vi "Check Stream Status.vi"(0 "niUsrpRio Session":T1={"FPGA Interface"=refnum, "RIO Interface Number"=0, "Data Clock Rate"=0, "FPGA Data Clock Rate"=0, "Global Settings Register Bus"=refnum, "Radio 0 Settings Register Bus"=refnum, "Radio 1 Settings Register Bus"=refnum, "Radio Settings Bus Semaphore"=refnum, "DB Queues"=[], "Characterization Data Valid?"=FALSE, "EEPROM Header"={"Checksum"=0, "Product Code"=0, "Hardware Current Version"=0, "Hardware Oldest Compatible Version"=0, "EEPROM Map Current Version"=0, "EEPROM Map Oldest Compatible Version"=0, "User Password"="", "Pointer to Factory Header"=0, "Pointer to User Header"=0, "Recommended Interval"=0, "Number of Reserved Bytes"=9, "Number of Daughterboards"=0, "Daughterboard IDs"=[], "Daughterboard Serial Numbers"=[]}, "Device Data Header"={"Checksum"=0, "Number of Channels"=0, "Number of Gain Settings"=[], "Pointer to Characterization Data"=[], "Number of Reserved Bytes"=27, "Number of Frequencies"=[]}, "EEPROM Characterization Header"={"Checksum"=0, "Date"=timestamp(0 s since 1904-01-01), "Temperature"=0.0, "Misc. Info"="", "Pointer to Device Data Header"=0, "Number of Reserved Bytes"=28}, "Characterization Data"=[], "FPGA Current Version"=0, "FPGA Oldest Compatible Version"=0, "Fixed Logic Current Version"=0, "Fixed Logic Oldest Compatible Version"=0, "FPGA Radio Settings Bus Current Version"=0, "FPGA Radio Settings Bus Oldest Compatible Version"=0, "FPGA Board Config Current Version"=0, "FPGA Board Config Oldest Compatible Version"=0} {"FPGA Data Clock Rate" format="%#.3pHz"; "Data Clock Rate" format="%#.3pHz"; "Characterization Data"."Frequencies [Hz]" format="%#_6p"; "EEPROM Characterization Header"."Pointer to Device Data Header" format="%x"; "EEPROM Characterization Header"."Checksum" format="%x"; "Device Data Header"."Pointer to Characterization Data" format="%x"; "Device Data Header"."Checksum" format="%x"; "EEPROM Header"."Pointer to User Header" format="%x"; "EEPROM Header"."Pointer to Factory Header" format="%x"; "EEPROM Header"."Product Code" format="%x"; "EEPROM Header"."Checksum" format="%x"}, 1 "scope":string(combo)="rx", 11 "error in":errorcluster, 12 "reference frequency source":string(combo)="Internal" caption="Reference Frequency Source") -> (4 "niUsrpRio Session (out)":T1={"FPGA Interface"=refnum, "RIO Interface Number"=0, "Data Clock Rate"=0, "FPGA Data Clock Rate"=0, "Global Settings Register Bus"=refnum, "Radio 0 Settings Register Bus"=refnum, "Radio 1 Settings Register Bus"=refnum, "Radio Settings Bus Semaphore"=refnum, "DB Queues"=[], "Characterization Data Valid?"=FALSE, "EEPROM Header"={"Checksum"=0, "Product Code"=0, "Hardware Current Version"=0, "Hardware Oldest Compatible Version"=0, "EEPROM Map Current Version"=0, "EEPROM Map Oldest Compatible Version"=0, "User Password"="", "Pointer to Factory Header"=0, "Pointer to User Header"=0, "Recommended Interval"=0, "Number of Reserved Bytes"=9, "Number of Daughterboards"=0, "Daughterboard IDs"=[], "Daughterboard Serial Numbers"=[]}, "Device Data Header"={"Checksum"=0, "Number of Channels"=0, "Number of Gain Settings"=[], "Pointer to Characterization Data"=[], "Number of Reserved Bytes"=27, "Number of Frequencies"=[]}, "EEPROM Characterization Header"={"Checksum"=0, "Date"=timestamp(0 s since 1904-01-01), "Temperature"=0.0, "Misc. Info"="", "Pointer to Device Data Header"=0, "Number of Reserved Bytes"=28}, "Characterization Data"=[], "FPGA Current Version"=0, "FPGA Oldest Compatible Version"=0, "Fixed Logic Current Version"=0, "Fixed Logic Oldest Compatible Version"=0, "FPGA Radio Settings Bus Current Version"=0, "FPGA Radio Settings Bus Oldest Compatible Version"=0, "FPGA Board Config Current Version"=0, "FPGA Board Config Oldest Compatible Version"=0} {"FPGA Data Clock Rate" format="%#.3pHz"; "Data Clock Rate" format="%#.3pHz"; "Characterization Data"."Frequencies [Hz]" format="%#_6p"; "EEPROM Characterization Header"."Pointer to Device Data Header" format="%x"; "EEPROM Characterization Header"."Checksum" format="%x"; "Device Data Header"."Pointer to Characterization Data" format="%x"; "Device Data Header"."Checksum" format="%x"; "EEPROM Header"."Pointer to User Header" format="%x"; "EEPROM Header"."Pointer to Factory Header" format="%x"; "EEPROM Header"."Product Code" format="%x"; "EEPROM Header"."Checksum" format="%x"}, 6 "done":bool caption="Done", 15 "error out":errorcluster)   [LabVIEW 2015]
doc: "Checks the status of the stream for when it is done, for FIFO overflows, for FIFO underflows, for DSP overflows, and if the clocks ever became unlocked. Checks the stream status after each Fetch Rx Data/Write Tx Data.\n\n<B>Input Parameters</B>\n\n<B>niUsrpRio Session</B> is the object created by the Open VI and used as the session handle for the USRP RIO design library.\n\n<B>Reference Frequency Source</B> is used when the source is GPS to determine whether to check whether the GPS became unlocked.\n\n<B>scope</B> is the channel to check the stream status. The options are \"rx/RF 0\", \"rx/RF 1\", \"tx/RF 0\", and \"tx/RF 1\".\n\n<B>error in</B> describes error conditions that occur before this node runs. This input provides standard 'error in' functionality.\n\n<B>Output Parameters</B>\n\n<B>niUsrpRio Session (out)</B> is the niUsrpRio session used in all subsequent USRP RIO design library host VIs.\n\n<B>Done</B> indicates when the acquisition/generation has completed.\n\n<B>error out</B> contains error information. This output provides standard 'error out' functionality."
uses:
  <instrlib>/niUsrpRio/Config/v1/Host/Public/niUsrpRio Session.ctl
  <instrlib>/_niInstr/Register Bus/v0/Host/Public/Register Bus Session.ctl
  <instrlib>/_niInstr/Register Bus/v0/Host/Private/Session Data.ctl
  <instrlib>/niUsrpRio/Config/v1/Host/Private/DB Queue Reference.ctl
  <instrlib>/niUsrpRio/Config/v1/Host/Private/Daughterboard Data.ctl
  <instrlib>/niUsrpRio/Config/v1/Host/Private/ATR state data.ctl
  <instrlib>/niUsrpRio/Config/v1/Host/Public/EEPROM Header.ctl
  <instrlib>/niUsrpRio/Config/v1/Host/Public/EEPROM Device Data Header.ctl
  <instrlib>/niUsrpRio/Config/v1/Host/Public/EEPROM Characterization Header.ctl
  <instrlib>/niUsrpRio/Config/v1/Host/Public/Characterization Data.ctl
  <instrlib>/niUsrpRio/Config/v1/Host/Public/IQ Imbalance.ctl
  FPGA/SubVIs/Stream Control State.ctl
  Streaming Xvcr FPGA Ref.ctl
  <instrlib>/niUsrpRio/Config/v1/Host/Public/What to Query for.ctl
  <vilib>/rvi/errors/niLvFpgaAdjustHostInterfaceError.vi
  <vilib>/rvi/interface/nirviReadWriteControl/nirviReadWriteControl.xnode
  NiFpgaLv.dll
  <vilib>/rvi/interface/Simulation/niFpgaSimulationCallBeginRW.vi
  <instrlib>/niUsrpRio/Config/v1/Host/niUsrpRio Config v1 Host.lvlib
  <instrlib>/_niInstr/Register Bus/v0/Host/niInstr Register Bus v0 Host.lvlib
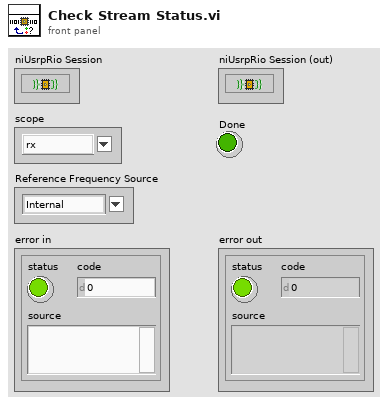
[diagram p1: front panel]
types:
  T1 = typedef "niUsrpRio Config v1 Host.lvlib/niUsrpRio Session.ctl" = cluster{"FPGA Interface":refnum<k20>, "RIO Interface Number":u32, "Data Clock Rate":u32, "FPGA Data Clock Rate":u32, "Global Settings Register Bus":T2, "Radio 0 Settings Register Bus":T2, "Radio 1 Settings Register Bus":T2, "Radio Settings Bus Semaphore":T3, "DB Queues":T4[], "Characterization Data Valid?":bool, "EEPROM Header":T5, "Device Data Header":T6, "EEPROM Characterization Header":T7, "Characterization Data":T8[], "FPGA Current Version":u32, "FPGA Oldest Compatible Version":u32, "Fixed Logic Current Version":u32, "Fixed Logic Oldest Compatible Version":u32, "FPGA Radio Settings Bus Current Version":u32, "FPGA Radio Settings Bus Oldest Compatible Version":u32, "FPGA Board Config Current Version":u32, "FPGA Board Config Oldest Compatible Version":u32}
  T2 = typedef "niInstr Register Bus v0 Host.lvlib/Register Bus Session.ctl" = refnum<queue>
  T3 = typedef "Semaphore RefNum" = refnum<k1>
  T4 = typedef "niUsrpRio Config v1 Host.lvlib/DB Queue Reference.ctl" = refnum<queue>
  T5 = typedef "niUsrpRio Config v1 Host.lvlib/EEPROM Header.ctl" = cluster{"Checksum":u32, "Product Code":u16, "Hardware Current Version":u16, "Hardware Oldest Compatible Version":u16, "EEPROM Map Current Version":u16, "EEPROM Map Oldest Compatible Version":u16, "User Password":string, "Pointer to Factory Header":u32, "Pointer to User Header":u32, "Recommended Interval":u16, "Number of Reserved Bytes":i32, "Number of Daughterboards":u8, "Daughterboard IDs":u16[], "Daughterboard Serial Numbers":string[]}
  T6 = typedef "niUsrpRio Config v1 Host.lvlib/EEPROM Device Data Header.ctl" = cluster{"Checksum":u32, "Number of Channels":u8, "Number of Gain Settings":u16[], "Pointer to Characterization Data":u32[], "Number of Reserved Bytes":i32, "Number of Frequencies":u16[]}
  T7 = typedef "niUsrpRio Config v1 Host.lvlib/EEPROM Characterization Header.ctl" = cluster{"Checksum":u32, "Date":timestamp, "Temperature":sgl, "Misc. Info":string, "Pointer to Device Data Header":u32, "Number of Reserved Bytes":i32}
  T8 = typedef "niUsrpRio Config v1 Host.lvlib/Characterization Data.ctl" = cluster{"Gains[dB]":dbl[], "Frequencies [Hz]":dbl[], "IQ Imbalance Table":T9[], "Measured Gains[dB]":dbl[][]}
  T9 = typedef "niUsrpRio Config v1 Host.lvlib/IQ Imbalance.ctl" = cluster{"Gain Imbalance [linear]":dbl, "Phase Imbalance [radians]":dbl, "Offset":cdb}
  T10 = typedef "niUsrpRio Config v1 Host.lvlib/What to Query for.ctl" = enum16{"Clock Chip Lock Status", "Clock Chip Ever Unlocked", "LO Lock Status", "GPS Lock Status", "GPS Ever Unlocked", "DRAM Ready Status", "DAC PLL Lock Status", "DAC Sync Lock Status", "Data Clock PLL Lock Status", "Data Clock PLL Ever Unlocked", "ADC Clock PLL Lock Status", "ADC Clock PLL Ever Unlocked", "ADC Data Valid Status", "ADC Data Ever Invalid"}
  T11 = typedef "Streaming Xvcr FPGA Ref.ctl" = refnum<k20>
  T12 = typedef "Stream Control State.ctl" = enum16{"Idle", "Active"}
  T13 = typedef "niUsrpRio Config v1 Host.lvlib/Device Subfunction.ctl" = enum16{"rx", "tx", "all"}
  T14 = typedef "niUsrpRio Config v1 Host.lvlib/RF Channel.ctl" = enum16{"0", "1", "All"}
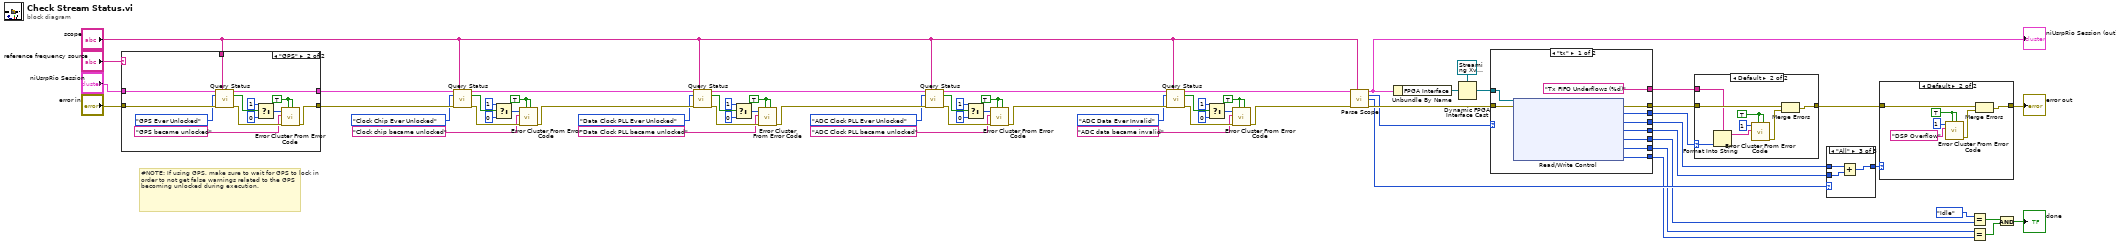
[diagram p0: block diagram]
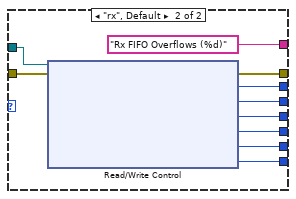
[diagram p7: hidden frame]
diagram:
  w12 = TRUE ("show call chain? (False)")
  w21 = TRUE ("show call chain? (False)")
  w26 = TRUE ("show call chain? (False)")
  w35 = TRUE ("show call chain? (False)")
  # "#NOTE: If using GPS, make sure to wait for GPS to lock in order to not get false warnings related to the GPS becoming unlocked during execution."
  n1 = case shown="\"GPS\"" "reference frequency source" {
    tunnel: "error in" -> [w69 w83]
    tunnel: "scope" -> [_ w71]
    tunnel: "niUsrpRio Session" -> [w70 w74]
    tunnel: [w70 w73] -> w7
    tunnel: [w69 w72] -> w68
    frame Default {
    }
    frame "GPS" {
      w79 = TRUE ("show call chain? (False)")
      n2 = call <instrlib>:"Query Status.vi"("niUsrpRio Session"=w74, "scope"=w71, "What to Query for"=What_to_Query_for."GPS Ever Unlocked", "error in"=w83) -> ("niUsrpRio Session (out)"=w73:T1, "Status"=w78:bool, "error out"=w82:errorcluster)  [unwired: 9 in]
      n3 = Select(t=1 ("error code (0)"), s=w78, f=0) -> (s? t:f=w77:i32)
      n4 = call <vilib>:"Error Cluster From Error Code.vi"("is warning? (False)"=w79, "show call chain? (False)"=w79, "error in (no error)"=w82, "error message (\"\")"="GPS became unlocked" ("error message (\"\")"), "error code (0)"=w77) -> ("error out"=w72:errorcluster)  [unwired: 4 in]
    }
  }
  n5 = call <instrlib>:"Query Status.vi"("niUsrpRio Session"=w7, "scope"="scope", "What to Query for"=What_to_Query_for."Clock Chip Ever Unlocked", "error in"=w68) -> ("niUsrpRio Session (out)"=w6:T1, "Status"=w34:bool, "error out"=w61:errorcluster)  [unwired: 9 in]
  n6 = Select(t=1 ("error code (0)"), s=w34, f=0) -> (s? t:f=w33:i32)
  n7 = call <vilib>:"Error Cluster From Error Code.vi"("is warning? (False)"=w35, "show call chain? (False)"=w35, "error in (no error)"=w61, "error message (\"\")"="Clock chip became unlocked" ("error message (\"\")"), "error code (0)"=w33) -> ("error out"=w67:errorcluster)  [unwired: 4 in]
  n8 = call <instrlib>:"Query Status.vi"("niUsrpRio Session"=w6, "scope"="scope", "What to Query for"=What_to_Query_for."Data Clock PLL Ever Unlocked", "error in"=w67) -> ("niUsrpRio Session (out)"=w5:T1, "Status"=w27:bool, "error out"=w64:errorcluster)  [unwired: 9 in]
  n9 = Select(t=1 ("error code (0)"), s=w27, f=0) -> (s? t:f=w28:i32)
  n10 = call <vilib>:"Error Cluster From Error Code.vi"("is warning? (False)"=w26, "show call chain? (False)"=w26, "error in (no error)"=w64, "error message (\"\")"="Data Clock PLL became unlocked" ("error message (\"\")"), "error code (0)"=w28) -> ("error out"=w66:errorcluster)  [unwired: 4 in]
  n11 = call <instrlib>:"Query Status.vi"("niUsrpRio Session"=w5, "scope"="scope", "What to Query for"=What_to_Query_for."ADC Clock PLL Ever Unlocked", "error in"=w66) -> ("niUsrpRio Session (out)"=w4:T1, "Status"=w20:bool, "error out"=w63:errorcluster)  [unwired: 9 in]
  n12 = Select(t=1 ("error code (0)"), s=w20, f=0) -> (s? t:f=w19:i32)
  n13 = call <vilib>:"Error Cluster From Error Code.vi"("is warning? (False)"=w21, "show call chain? (False)"=w21, "error in (no error)"=w63, "error message (\"\")"="ADC Clock PLL became unlocked" ("error message (\"\")"), "error code (0)"=w19) -> ("error out"=w65:errorcluster)  [unwired: 4 in]
  n14 = call <instrlib>:"Query Status.vi"("niUsrpRio Session"=w4, "scope"="scope", "What to Query for"=What_to_Query_for."ADC Data Ever Invalid", "error in"=w65) -> ("niUsrpRio Session (out)"=w3:T1, "Status"=w13:bool, "error out"=w62:errorcluster)  [unwired: 9 in]
  n15 = Select(t=1 ("error code (0)"), s=w13, f=0) -> (s? t:f=w14:i32)
  n16 = call <vilib>:"Error Cluster From Error Code.vi"("is warning? (False)"=w12, "show call chain? (False)"=w12, "error in (no error)"=w62, "error message (\"\")"="ADC data became invalid" ("error message (\"\")"), "error code (0)"=w14) -> ("error out"=w2:errorcluster)  [unwired: 4 in]
  n17 = call <instrlib>:"Parse Scope.vi"("niUsrpRio Session"=w3, "scope"="scope", "error in"=w2) -> ("niUsrpRio Session (out)"=w56:T1, "Device Subfunction"=w55:T13, "Device Subfunction Channel"=w48:T14, "error out"=w60:errorcluster)  [unwired: 4 in, 5 out]
  "niUsrpRio Session (out)" <- w56
  n18 = Unbundle By Name(w56) -> ("FPGA Interface"=w40:refnum<k20>)
  n19 = Dynamic FPGA Interface Cast(Session In=T11 refnum ("USRP RIO Streaming Xcvr FPGA VI Reference"), Type=w40) -> (Session Out=w39:T11)
  n20 = case shown="\"tx\"" w55 {
    tunnel: w60 -> [w93 w103]
    tunnel: [w92 w102] -> w53
    tunnel: [w91 w101] -> w54
    tunnel: [w90 w100] -> w50
    tunnel: [w89 w99] -> w49
    tunnel: [w88 w98] -> w46
    tunnel: [w87 w97] -> w45
    tunnel: [w86 w96] -> w44
    tunnel: ["Tx FIFO Underflows (%d)" ("error message (\"\")") "Rx FIFO Overflows (%d)" ("error message (\"\")")] -> w52
    tunnel: w39 -> [w84 w94]
    frame "tx" {
      n21 = xnode "Read/Write Control"("FPGA VI Reference In"=w84, "error in"=w93) -> ("error out"=w91:errorcluster, "tx.number of fifo underflows"=w92:u32, "tx 0.number of IQ data overflows"=w90:u64, "tx 1.number of IQ data overflows"=w89:u64, "tx.state"=w88:enum16{"Idle", "Active"}, "tx.samples processed"=w87:u32, "tx.samples to generate"=w86:u32)  [unwired: 1 out]
    }
    frame "rx", Default {
      n22 = xnode "Read/Write Control"("FPGA VI Reference In"=w94, "error in"=w103) -> ("error out"=w101:errorcluster, "rx.number of fifo overflows"=w102:u32, "rx 0.number of IQ data overflows"=w100:u64, "rx 1.number of IQ data overflows"=w99:u64, "rx.state"=w98:enum16{"Idle", "Active"}, "rx.samples processed"=w97:u32, "rx.samples to acquire"=w96:u32)  [unwired: 1 out]
    }
  }
  n23 = case shown="Default" w53 {
    selector: w53 -> [_ w106]
    tunnel: w54 -> [w104 w111]
    tunnel: [w104 w109] -> w51
    tunnel: w52 -> [_ w105]
    frame 0 {
    }
    frame Default {
      w107 = TRUE ("show call chain? (False)")
      n24 = Format Into String(format string=w105, w106) -> (resulting string=w108:string)  [unwired: 2 in, 1 out]
      n25 = call <vilib>:"Error Cluster From Error Code.vi"("is warning? (False)"=w107, "show call chain? (False)"=w107, "error message (\"\")"=w108, "error code (0)"=1) -> ("error out"=w110:errorcluster)  [unwired: 5 in]
      n26 = Merge Errors(w111, w110) -> (w109:errorcluster)
    }
  }
  n27 = case shown="\"All\"" w48 {
    tunnel: w50 -> [w113 _ w117]
    tunnel: w49 -> [_ w114 w116]
    tunnel: [w113 w114 w115] -> w47
    frame "0", Default {
    }
    frame "1" {
    }
    frame "All" {
      n28 = Add(x=w117, y=w116) -> (x+y=w115:u64)
    }
  }
  n29 = case shown="Default" w47 {
    tunnel: w51 -> [w118 w122]
    tunnel: [w118 w120] -> w42
    frame 0 {
    }
    frame Default {
      w119 = TRUE ("show call chain? (False)")
      n30 = call <vilib>:"Error Cluster From Error Code.vi"("is warning? (False)"=w119, "show call chain? (False)"=w119, "error message (\"\")"="DSP Overflow" ("error message (\"\")"), "error code (0)"=1) -> ("error out"=w121:errorcluster)  [unwired: 5 in]
      n31 = Merge Errors(w122, w121) -> (w120:errorcluster)
    }
  }
  "error out" <- w42
  n32 = Equal?(x=Stream_Control_State."Idle" ("state"), y=w46) -> (x = y?=w59:bool)
  n33 = Equal?(x=w45, y=w44) -> (x = y?=w58:bool)
  n34 = And(x=w59, y=w58) -> (x .and. y?=→"done":bool)
